vi "m1m3_logEvent_ForceActuatorWarning.vi"(8 "error in (no error)":errorcluster, 11 "logevent_ForceActuatorWarning_Ctl":T1) -> (0 "error out":errorcluster, 2 "function return":i32, 3 "logevent_ForceActuatorWarning_Ctl out":T1)   [LabVIEW 2016, in "SALLV_m1m3.lvlib"]
doc: "int m1m3_shm_logEvent_ForceActuatorWarningLV(m1m3_logevent_ForceActuatorWarningLV *logevent_ForceActuatorWarning_Ctl );"
uses:
  SALLV_m1m3.lvlib
  DataTypes/logevent_ForceActuatorWarning.ctl
  SALLV_m1m3.so
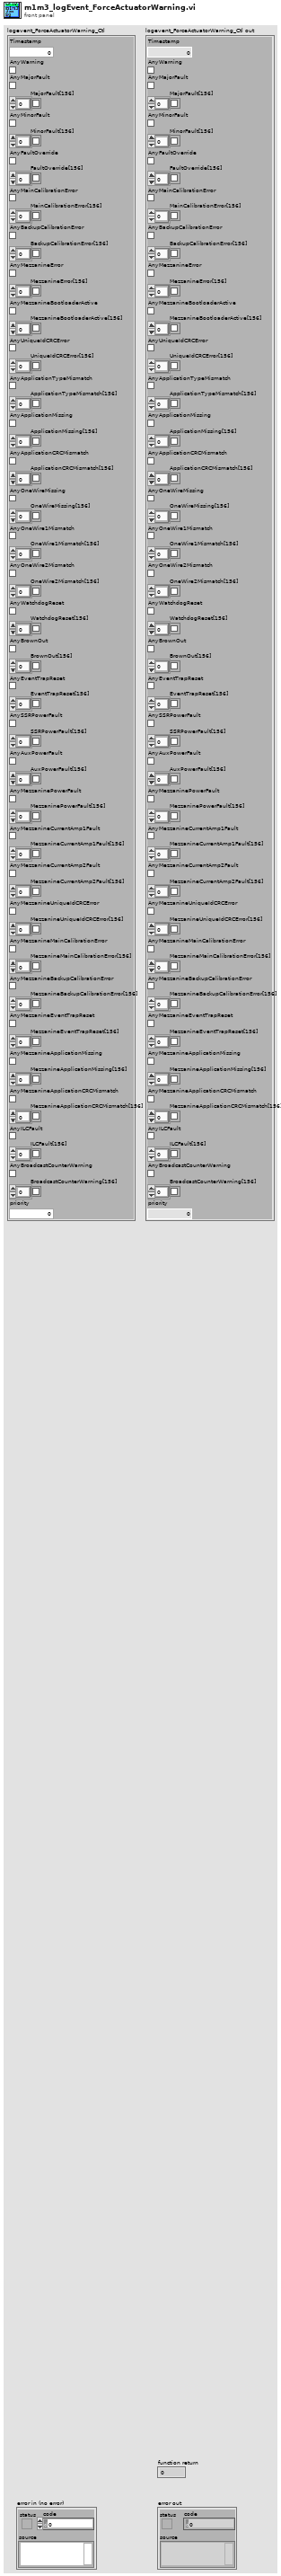
[diagram p1: front panel]
types:
  T1 = typedef "SALLV_m1m3.lvlib/logevent_ForceActuatorWarning.ctl" = cluster{"Timestamp":dbl, "AnyWarning":bool, "AnyMajorFault":bool, "MajorFault[156]":bool[], "AnyMinorFault":bool, "MinorFault[156]":bool[], "AnyFaultOverride":bool, "FaultOverride[156]":bool[], "AnyMainCalibrationError":bool, "MainCalibrationError[156]":bool[], "AnyBackupCalibrationError":bool, "BackupCalibrationError[156]":bool[], "AnyMezzanineError":bool, "MezzanineError[156]":bool[], "AnyMezzanineBootloaderActive":bool, "MezzanineBootloaderActive[156]":bool[], "AnyUniqueIdCRCError":bool, "UniqueIdCRCError[156]":bool[], "AnyApplicationTypeMismatch":bool, "ApplicationTypeMismatch[156]":bool[], "AnyApplicationMissing":bool, "ApplicationMissing[156]":bool[], "AnyApplicationCRCMismatch":bool, "ApplicationCRCMismatch[156]":bool[], "AnyOneWireMissing":bool, "OneWireMissing[156]":bool[], "AnyOneWire1Mismatch":bool, "OneWire1Mismatch[156]":bool[], "AnyOneWire2Mismatch":bool, "OneWire2Mismatch[156]":bool[], "AnyWatchdogReset":bool, "WatchdogReset[156]":bool[], "AnyBrownOut":bool, "BrownOut[156]":bool[], "AnyEventTrapReset":bool, "EventTrapReset[156]":bool[], "AnySSRPowerFault":bool, "SSRPowerFault[156]":bool[], "AnyAuxPowerFault":bool, "AuxPowerFault[156]":bool[], "AnyMezzaninePowerFault":bool, "MezzaninePowerFault[156]":bool[], "AnyMezzanineCurrentAmp1Fault":bool, "MezzanineCurrentAmp1Fault[156]":bool[], "AnyMezzanineCurrentAmp2Fault":bool, "MezzanineCurrentAmp2Fault[156]":bool[], "AnyMezzanineUniqueIdCRCError":bool, "MezzanineUniqueIdCRCError[156]":bool[], "AnyMezzanineMainCalibrationError":bool, "MezzanineMainCalibrationError[156]":bool[], "AnyMezzanineBackupCalibrationError":bool, "MezzanineBackupCalibrationError[156]":bool[], "AnyMezzanineEventTrapReset":bool, "MezzanineEventTrapReset[156]":bool[], "AnyMezzanineApplicationMissing":bool, "MezzanineApplicationMissing[156]":bool[], "AnyMezzanineApplicationCRCMismatch":bool, "MezzanineApplicationCRCMismatch[156]":bool[], "AnyILCFault":bool, "ILCFault[156]":bool[], "AnyBroadcastCounterWarning":bool, "BroadcastCounterWarning[156]":bool[], "priority":i32}
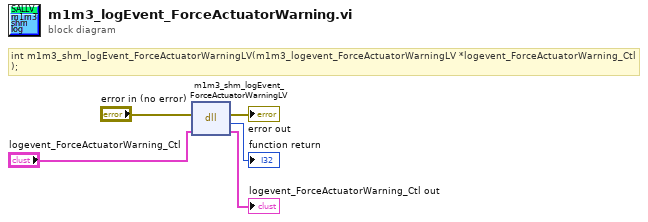
[diagram p0: block diagram]
diagram:
  # "int m1m3_shm_logEvent_ForceActuatorWarningLV(m1m3_logevent_ForceActuatorWarningLV *logevent_ForceActuatorWarning_Ctl );"
  n1 = dll-call lib="opt/CODE/SALLV_m1m3/SALLV_m1m3.*" fn="m1m3_shm_logEvent_ForceActuatorWarningLV"(error in="error in (no error)", "logevent_ForceActuatorWarning_Ctl"="logevent_ForceActuatorWarning_Ctl") -> (error out=→"error out":errorcluster, →"function return":i32, "logevent_ForceActuatorWarning_Ctl"=→"logevent_ForceActuatorWarning_Ctl out":T1)  [unwired: 2 in, 1 out]
